vi "niScope Mux Open.vi"(8 "error in":errorcluster, 11 "adc session in":T2={"niScope"={"channel cfg"=[], "sessions"=[], "multi cards"=FALSE, "channels"=0, "type"=enum."n/a", "memory [B/chn]"=0, "ext. clock [Hz]"=0.0, "samples count"=0, "use streaming"=FALSE, "proc setup"={"packet size [smpl]"=0, "current timeout [s]"=0.0, "blk2blk timeout [s]"=0.0, "event time"=timestamp(0 s since 1904-01-01), "temp sampl T [s]"=0.0, "data queue"=refnum, "stop notifier"=refnum, "proc ref"=refnum}, "sample width [B]"=0, "ranges [V]"=[], "trigger setup"={"coupling"=1, "level [V]"=0.0, "slope"=0, "mode"=enum."Immediate"}, "fs [Hz]"=0.0, "bitres [bit]"=0, "clock source"=enum."VAL_NO_SOURCE"}, "3458A"={"channels"=[], "sync unit"={"VISA"="", "type"=enum."Picotest U6200A"}, "awg unit"={"type"=enum."Agilent 331xxA to 332xxA", "VISA"="", "enable 10MHz ref"=FALSE}, "sync mode"=enum."MASTER-SLAVE, MASTER clocked by TIMER", "streaming mode"=FALSE, "idn mode"=enum."Auto", "sampling mode"=enum."DCV", "Ts [s]"=0.0, "sample memory [B]"=0, "proc setup"={"channel id"=0, "packet size [smpl]"=0, "current timeout [s]"=0.0, "blk2blk timeout [s]"=0.0, "event time"=timestamp(0 s since 1904-01-01), "stop notifier"=refnum, "data queues"=[], "proc refs"=[], "bus semaphore"=refnum}, "sample size [B]"=0, "sample count"=0, "aux data"={"channel id"=0, "valid?"=[], "gain [V]"=[], "timestamp [s]"=[], "Ts [s]"=0.0, "abs timestamp"=timestamp(0 s since 1904-01-01), "t [deg C]"=[], "multiplex timestamp [s]"=-1.0, "only multiplex?"=FALSE, "multiplex smpl offset"=0}, "ranges [V]"=[], "aperture [s]"=0.0, "LEVEL trigger"={"edge"=enum."POS", "level [V]"=0.0, "coupling"=enum."DC"}, "trigger mode"=enum."AUTO", "measure temp.?"=FALSE, "disp mesages"=[], "shared bus?"=FALSE, "disable display?"=FALSE, "aper mode"=enum."Manual", "aper rules"=[], "multiplex"={"cycles"=0, "delay [s]"=0.0, "enabled"=FALSE, "overhead [s]"=1.0, "tot smpls"=0}}, "dsdll"={"dsdll"={"dsdll path"=path "", "dsdll handle"=[], "output devices"=[], "capture devices"=[]}, "channels"=0, "device id"=0, "channel idns"=[], "proc setup"={"packet size [smpl]"=0, "current timeout [s]"=0.0, "blk2blk timeout [s]"=0.0, "event time"=timestamp(0 s since 1904-01-01), "data queue"=refnum, "stop notifier"=refnum, "proc ref"=refnum}, "samples count"=0, "fs [Hz]"=0.0}, "type"=enum."niScope", "channel idn str"=[], "aux instr idn str"=[], "modified?"=FALSE, "simadc"={"channels"=[], "range [V]"=0.0, "Ts step [s]"=0.0, "time [s]"=0.0, "fs [Hz]"=0.0, "count"=0, "smpl offset"=0, "set count"=0, "bit res"=0}, "force rst?"=FALSE, "exit mode"=enum."Immediate reset", "exit dly"=0.0, "exit tmr"=timestamp(0 s since 1904-01-01), "busy?"=FALSE, "accessed?"=FALSE, "multiplex"={"Type"=enum."Dummy", "gen com ssn"={"visa"="", "primary"=enum."None", "secondary"=enum."None", "channels"=[]}, "delay before [s]"=0.0, "delay post [s]"=0.0, "sequence"=[], "enabled"=FALSE, "ref timestamp [s]"=0.0, "idn string"="", "dev niScope"="", "niScope idx"=0}} {"3458A"."channels"."Range [Vpk]" min=0.0; "niScope"."trigger setup"."level [V]" format="%.2f"; "niScope"."trigger setup"."coupling" items=["AC"=0, "DC"=1, "HF Reject"=3, "LF Reject"=4, "AC Plus HF Reject"=1001]; "niScope"."channel cfg"."Range [Vpk]" min=0.0; "niScope"."channel cfg"."Channel" min=0}) -> (0 "error out":errorcluster, 2 "idn string":string, 3 "adc session out":T2={"niScope"={"channel cfg"=[], "sessions"=[], "multi cards"=FALSE, "channels"=0, "type"=enum."n/a", "memory [B/chn]"=0, "ext. clock [Hz]"=0.0, "samples count"=0, "use streaming"=FALSE, "proc setup"={"packet size [smpl]"=0, "current timeout [s]"=0.0, "blk2blk timeout [s]"=0.0, "event time"=timestamp(0 s since 1904-01-01), "temp sampl T [s]"=0.0, "data queue"=refnum, "stop notifier"=refnum, "proc ref"=refnum}, "sample width [B]"=0, "ranges [V]"=[], "trigger setup"={"coupling"=1, "level [V]"=0.0, "slope"=0, "mode"=enum."Immediate"}, "fs [Hz]"=0.0, "bitres [bit]"=0, "clock source"=enum."VAL_NO_SOURCE"}, "3458A"={"channels"=[], "sync unit"={"VISA"="", "type"=enum."Picotest U6200A"}, "awg unit"={"type"=enum."Agilent 331xxA to 332xxA", "VISA"="", "enable 10MHz ref"=FALSE}, "sync mode"=enum."MASTER-SLAVE, MASTER clocked by TIMER", "streaming mode"=FALSE, "idn mode"=enum."Auto", "sampling mode"=enum."DCV", "Ts [s]"=0.0, "sample memory [B]"=0, "proc setup"={"channel id"=0, "packet size [smpl]"=0, "current timeout [s]"=0.0, "blk2blk timeout [s]"=0.0, "event time"=timestamp(0 s since 1904-01-01), "stop notifier"=refnum, "data queues"=[], "proc refs"=[], "bus semaphore"=refnum}, "sample size [B]"=0, "sample count"=0, "aux data"={"channel id"=0, "valid?"=[], "gain [V]"=[], "timestamp [s]"=[], "Ts [s]"=0.0, "abs timestamp"=timestamp(0 s since 1904-01-01), "t [deg C]"=[], "multiplex timestamp [s]"=-1.0, "only multiplex?"=FALSE, "multiplex smpl offset"=0}, "ranges [V]"=[], "aperture [s]"=0.0, "LEVEL trigger"={"edge"=enum."POS", "level [V]"=0.0, "coupling"=enum."DC"}, "trigger mode"=enum."AUTO", "measure temp.?"=FALSE, "disp mesages"=[], "shared bus?"=FALSE, "disable display?"=FALSE, "aper mode"=enum."Manual", "aper rules"=[], "multiplex"={"cycles"=0, "delay [s]"=0.0, "enabled"=FALSE, "overhead [s]"=1.0, "tot smpls"=0}}, "dsdll"={"dsdll"={"dsdll path"=path "", "dsdll handle"=[], "output devices"=[], "capture devices"=[]}, "channels"=0, "device id"=0, "channel idns"=[], "proc setup"={"packet size [smpl]"=0, "current timeout [s]"=0.0, "blk2blk timeout [s]"=0.0, "event time"=timestamp(0 s since 1904-01-01), "data queue"=refnum, "stop notifier"=refnum, "proc ref"=refnum}, "samples count"=0, "fs [Hz]"=0.0}, "type"=enum."niScope", "channel idn str"=[], "aux instr idn str"=[], "modified?"=FALSE, "simadc"={"channels"=[], "range [V]"=0.0, "Ts step [s]"=0.0, "time [s]"=0.0, "fs [Hz]"=0.0, "count"=0, "smpl offset"=0, "set count"=0, "bit res"=0}, "force rst?"=FALSE, "exit mode"=enum."Immediate reset", "exit dly"=0.0, "exit tmr"=timestamp(0 s since 1904-01-01), "busy?"=FALSE, "accessed?"=FALSE, "multiplex"={"Type"=enum."Dummy", "gen com ssn"={"visa"="", "primary"=enum."None", "secondary"=enum."None", "channels"=[]}, "delay before [s]"=0.0, "delay post [s]"=0.0, "sequence"=[], "enabled"=FALSE, "ref timestamp [s]"=0.0, "idn string"="", "dev niScope"="", "niScope idx"=0}} {"3458A"."channels"."Range [Vpk]" min=0.0; "niScope"."trigger setup"."level [V]" format="%.2f"; "niScope"."trigger setup"."coupling" items=["AC"=0, "DC"=1, "HF Reject"=3, "LF Reject"=4, "AC Plus HF Reject"=1001]; "niScope"."channel cfg"."Range [Vpk]" min=0.0; "niScope"."channel cfg"."Channel" min=0})   [LabVIEW 2013]
doc: "This VI tries to open virtual digitizer channel for multiplexer control. It shares device session with digitizer, so correct use is:\n1) initialize digitizer\n2) call this VI\n3) do stuff\n4) close multiplexer\n3) close digitizer"
uses:
  adc/ADC Session.ctl
  niScope/niScope Session.ctl
  niScope/niScope Virtual Channel Config.ctl
  niScope/niScope Virtual Channel Mode.ctl
  niScope/niScope Virtual Channel Input Z.ctl
  niScope/niScope Virtual Channel Coupling.ctl
  niScope/niScope Type.ctl
  niScope/niScope Digitizing Process Options.ctl
  niScope/niScope Data Packet.ctl
  niScope/niScope Trigger Setup.ctl
  <instrlib>/niScope/Controls/niScope trigger coupling.ctl
  <instrlib>/niScope/Controls/niScope trigger slope.ctl
  niScope/niScope Reference Clock.ctl
  DMM/3458A Digitizer Session.ctl
  DMM/3458A Virtual Channel Config.ctl
  Counter/Counter Session.ctl
  Counter/Counter Type.ctl
  AWG/AWG Session.ctl
  AWG/AWG Type.ctl
  DMM/3458A Sync Mode.ctl
  DMM/3458A Idn Mode.ctl
  DMM/3458A Digitizing Low Levels/Configure/Sampling Mode.ctl
  DMM/3458A Digitizing Process Options.ctl
  DMM/3458A Data Packet.ctl
  DMM/3458A Aux Record Data.ctl
  DMM/3458A Digitizing Low Levels/Configure/Level Setup.ctl
  DMM/3458A Digitizing Low Levels/Configure/First Sample Trigger.ctl
  DMM/3458A Aperture Selection Mode.ctl
  DMM/3458A Multiplexing Config.ctl
  dsdll/DSDLL Session.ctl
  dsdll/dsdll.lvlibp/dsdll_instance.ctl
  dsdll/dsdll.lvlibp/dsdll_device_record.ctl
  dsdll/DSDLL Process Config.ctl
  dsdll/DSDLL Data Packet.ctl
  adc/ADC Type.ctl
  simulated_adc/SimAdc Config.ctl
  simulated_adc/SimAdc Channel Cfg.ctl
  adc/ADC On Close Action.ctl
  adc/Multiplexer/MPX Session.ctl
  adc/Multiplexer/MPX Type.ctl
  Generic COM/GCOMM Session.ctl
  Generic COM/GCOMM Signal.ctl
  Generic COM/GCOMM Virtual Channel.ctl
  Generic COM/GCOMM Logic State.ctl
  <vilib>/Utility/error.llb/Error Cluster From Error Code.vi
  <vilib>/ErrorRing/Error Ring.xnode
  niScope/niScope Virtual Digitizer.lvlib
  DMM/3458A Virtual Digitizer.lvlib
  Counter/Counter.lvlib
  AWG/AWG.lvlib
  DMM/3458A Digitizing Low Levels/3458A Digitizing Low Levels.lvlib
  dsdll/dsdll.lvlibp
  dsdll/DSDLL Virtual Digitizer.lvlib
panel:
  in  "type":T1
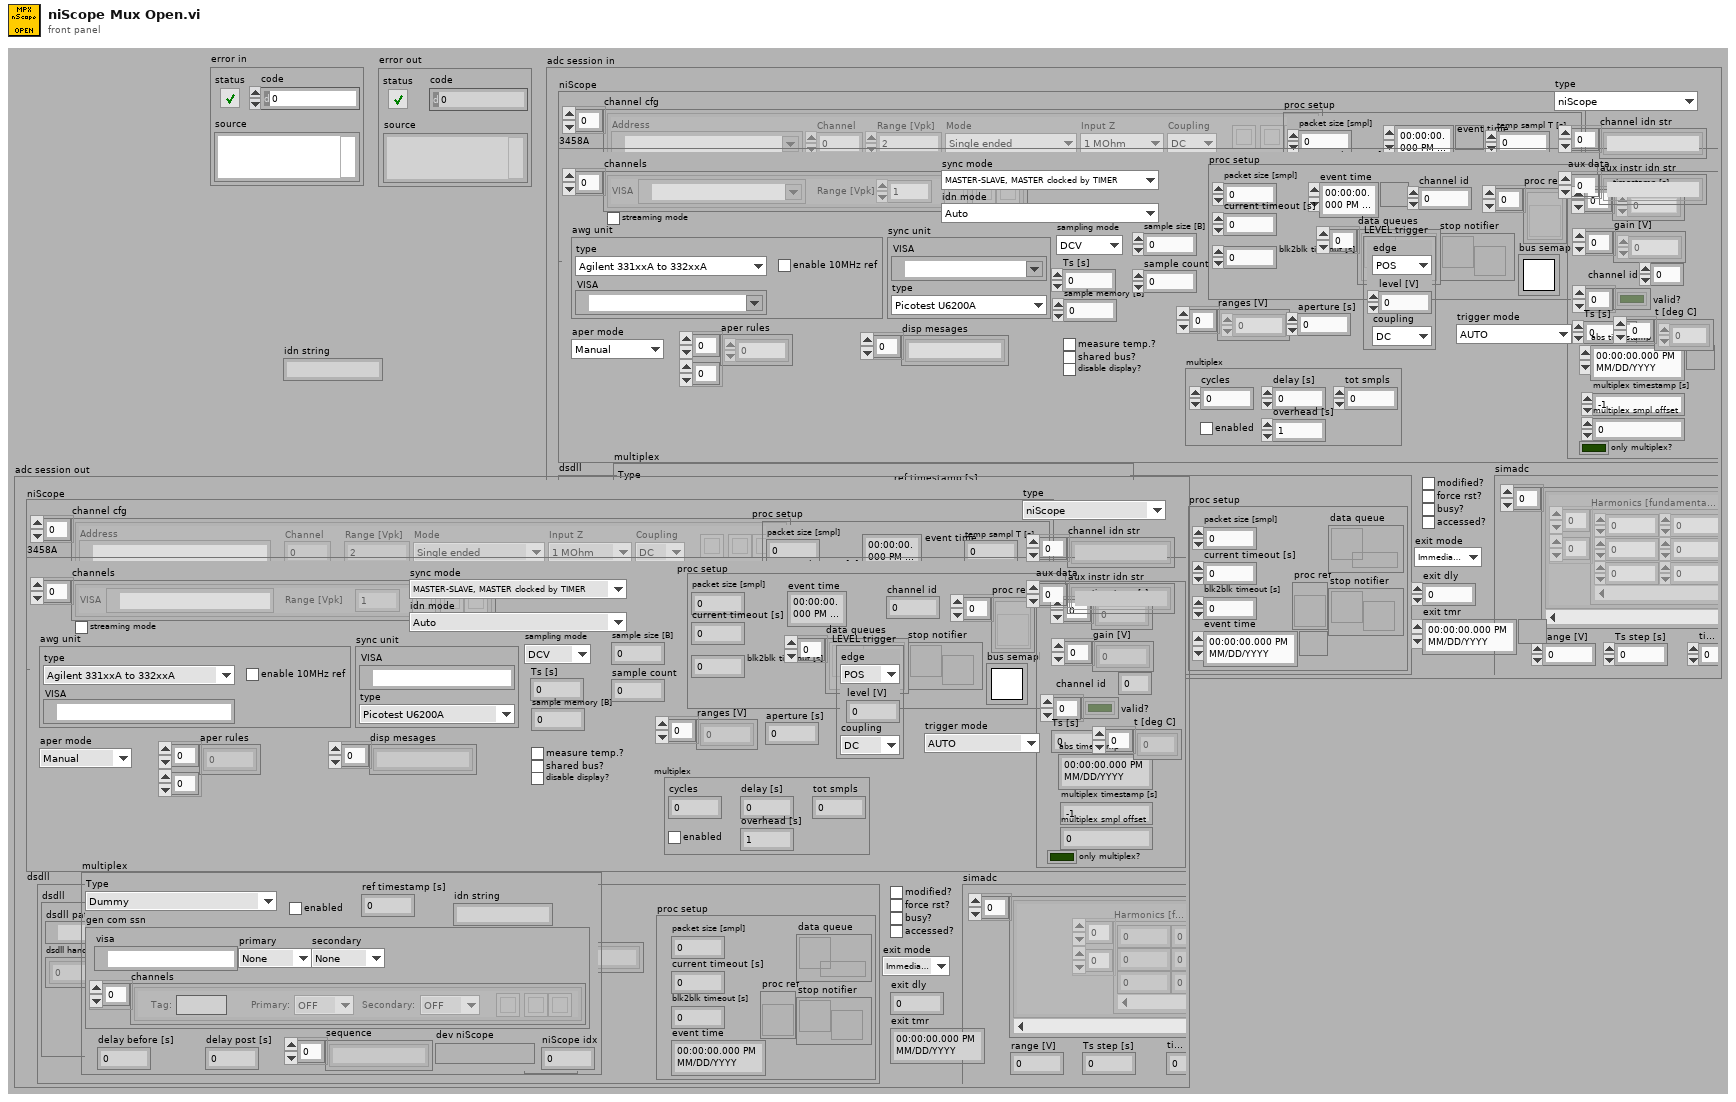
[diagram p1: front panel]
types:
  T1 = typedef "ADC Type.ctl" = enum16{"niScope", "3458A", "DirectSound DLL", "dummy"}
  T2 = typedef "ADC Session.ctl" = cluster{"niScope":T3, "3458A":T14, "dsdll":T30, "type":T1, "channel idn str":string[], "aux instr idn str":string[], "modified?":bool, "simadc":T34, "force rst?":bool, "exit mode":T36, "exit dly":dbl, "exit tmr":timestamp, "busy?":bool, "accessed?":bool, "multiplex":T37}
  T3 = typedef "niScope Virtual Digitizer.lvlib/niScope Session.ctl" = cluster{"channel cfg":T4[], "sessions":refnum<k20>[], "multi cards":bool, "channels":i32, "type":T8, "memory [B/chn]":i32, "ext. clock [Hz]":dbl, "samples count":i64, "use streaming":bool, "proc setup":T9, "sample width [B]":i32, "ranges [V]":dbl[], "trigger setup":T10, "fs [Hz]":dbl, "bitres [bit]":i32, "clock source":T13}
  T4 = typedef "niScope Virtual Digitizer.lvlib/niScope Virtual Channel Config.ctl" = cluster{"Address":refnum<k15>, "Channel":i32, "Mode":T5, "Input Z":T6, "Coupling":T7, "Range [Vpk]":dbl, "btn clr":bool, "btn up":bool, "btn down":bool}
  T5 = typedef "niScope Virtual Digitizer.lvlib/niScope Virtual Channel Mode.ctl" = enum16{"Single ended", "Unbal. differential", "Differential"}
  T6 = typedef "niScope Virtual Digitizer.lvlib/niScope Virtual Channel Input Z.ctl" = enum16{"1 MOhm", "50 Ohm"}
  T7 = typedef "niScope Virtual Digitizer.lvlib/niScope Virtual Channel Coupling.ctl" = enum16{"AC", "DC", "GND"}
  T8 = typedef "niScope Virtual Digitizer.lvlib/niScope Type.ctl" = enum16{"n/a", "5922"}
  T9 = typedef "niScope Virtual Digitizer.lvlib/niScope Digitizing Process Options.ctl" = cluster{"packet size [smpl]":i64, "current timeout [s]":dbl, "blk2blk timeout [s]":dbl, "event time":timestamp, "temp sampl T [s]":dbl, "data queue":refnum<queue>, "stop notifier":refnum<notifier>, "proc ref":refnum<vi>}
  T10 = typedef "niScope Virtual Digitizer.lvlib/niScope Trigger Setup.ctl" = cluster{"coupling":T11, "level [V]":dbl, "slope":T12, "mode":enum16{"Immediate", "External", "Level"}}
  T11 = typedef "niScope trigger coupling.ctl" = u16
  T12 = typedef "niScope trigger slope.ctl" = i32
  T13 = typedef "niScope Virtual Digitizer.lvlib/niScope Reference Clock.ctl" = enum16{"VAL_NO_SOURCE", "VAL_CLK_IN", "VAL_PXI_CLOCK", "VAL_EXTERNAL"}
  T14 = typedef "3458A Virtual Digitizer.lvlib/3458A Digitizer Session.ctl" = cluster{"channels":T15[], "sync unit":T16, "awg unit":T18, "sync mode":T20, "streaming mode":bool, "idn mode":T21, "sampling mode":T22, "Ts [s]":dbl, "sample memory [B]":i32, "proc setup":T23, "sample size [B]":i32, "sample count":i32, "aux data":T25, "ranges [V]":dbl[], "aperture [s]":dbl, "LEVEL trigger":T26, "trigger mode":T27, "measure temp.?":bool, "disp mesages":string[], "shared bus?":bool, "disable display?":bool, "aper mode":T28, "aper rules":dbl[][], "multiplex":T29}
  T15 = typedef "3458A Virtual Digitizer.lvlib/3458A Virtual Channel Config.ctl" = cluster{"VISA":refnum<visa-resource-name>, "Range [Vpk]":dbl, "btn clr":bool, "btn up":bool, "btn down":bool}
  T16 = typedef "Counter.lvlib/Counter Session.ctl" = cluster{"VISA":refnum<visa-resource-name>, "type":T17}
  T17 = typedef "Counter.lvlib/Counter Type.ctl" = enum16{"Picotest U6200A", "dummy"}
  T18 = typedef "AWG.lvlib/AWG Session.ctl" = cluster{"type":T19, "VISA":refnum<visa-resource-name>, "enable 10MHz ref":bool}
  T19 = typedef "AWG.lvlib/AWG Type.ctl" = enum16{"Agilent 331xxA to 332xxA", "Agilent 335xxA to 336xxA", "Tektronix AFG3101C", "dummy"}
  T20 = typedef "3458A Virtual Digitizer.lvlib/3458A Sync Mode.ctl" = enum16{"MASTER-SLAVE, MASTER clocked by TIMER", "MASTER-SLAVE, MASTER clocked by AWG", "ALL clocked by AWG", "MASTER-SLAVE, ALL clocked by TIMER", "ALL clocked by AWG with DFLL"}
  T21 = typedef "3458A Virtual Digitizer.lvlib/3458A Idn Mode.ctl" = enum16{"Auto", "Sequential (chn A, chn B, ...)", "From calibration string"}
  T22 = typedef "3458A Virtual Digitizer.lvlib/3458A Digitizing Low Levels.lvlib/Sampling Mode.ctl" = enum16{"DCV", "DSDC", "DSAC"}
  T23 = typedef "3458A Virtual Digitizer.lvlib/3458A Digitizing Process Options.ctl" = cluster{"channel id":i32, "packet size [smpl]":i32, "current timeout [s]":dbl, "blk2blk timeout [s]":dbl, "event time":timestamp, "stop notifier":refnum<notifier>, "data queues":refnum<queue>[], "proc refs":refnum<vi>[], "bus semaphore":T24}
  T24 = typedef "Semaphore RefNum" = refnum<k1>
  T25 = typedef "3458A Virtual Digitizer.lvlib/3458A Aux Record Data.ctl" = cluster{"channel id":i32, "valid?":bool[], "gain [V]":dbl[], "timestamp [s]":dbl[], "Ts [s]":dbl, "abs timestamp":timestamp, "t [deg C]":dbl[], "multiplex timestamp [s]":dbl, "only multiplex?":bool, "multiplex smpl offset":i64}
  T26 = typedef "3458A Virtual Digitizer.lvlib/3458A Digitizing Low Levels.lvlib/Level Setup.ctl" = cluster{"edge":enum16{"POS", "NEG"}, "level [V]":dbl, "coupling":enum16{"DC", "AC"}}
  T27 = typedef "3458A Virtual Digitizer.lvlib/3458A Digitizing Low Levels.lvlib/First Sample Trigger.ctl" = enum16{"AUTO", "EXT", "SYN", "SGL", "HOLD", "LEVEL"}
  T28 = typedef "3458A Virtual Digitizer.lvlib/3458A Aperture Selection Mode.ctl" = enum16{"Manual", "Maximum", "Table"}
  T29 = typedef "3458A Multiplexing Config.ctl" = cluster{"cycles":i32, "delay [s]":dbl, "enabled":bool, "overhead [s]":dbl, "tot smpls":i64}
  T30 = typedef "DSDLL Virtual Digitizer.lvlib/DSDLL Session.ctl" = cluster{"dsdll":T31, "channels":i32, "device id":i32, "channel idns":string[], "proc setup":T33, "samples count":i32, "fs [Hz]":dbl}
  T31 = typedef "dsdll.lvlibp/dsdll_instance.ctl" = cluster{"dsdll path":path, "dsdll handle":u8[], "output devices":T32[], "capture devices":T32[]}
  T32 = typedef "dsdll.lvlibp/dsdll_device_record.ctl" = cluster{"guid":u8[], "name":string}
  T33 = typedef "DSDLL Virtual Digitizer.lvlib/DSDLL Process Config.ctl" = cluster{"packet size [smpl]":i32, "current timeout [s]":dbl, "blk2blk timeout [s]":dbl, "event time":timestamp, "data queue":refnum<queue>, "stop notifier":refnum<notifier>, "proc ref":refnum<vi>}
  T34 = typedef "SimAdc Config.ctl" = cluster{"channels":T35[], "range [V]":dbl, "Ts step [s]":dbl, "time [s]":dbl, "fs [Hz]":dbl, "count":i64, "smpl offset":i64, "set count":i64, "bit res":i32}
  T35 = typedef "SimAdc Channel Cfg.ctl" = cluster{"harmonics":dbl[][], "btn clear":bool, "noise":dbl, "fundamental [Hz]":dbl}
  T36 = typedef "ADC On Close Action.ctl" = enum16{"Immediate reset", "Delayed reset"}
  T37 = typedef "MPX Session.ctl" = cluster{"Type":T38, "gen com ssn":T39, "delay before [s]":dbl, "delay post [s]":dbl, "sequence":string[], "enabled":bool, "ref timestamp [s]":dbl, "idn string":string, "dev niScope":refnum<k15>, "niScope idx":i32}
  T38 = typedef "MPX Type.ctl" = enum16{"Dummy", "Generic - COM port", "Generic - niScope PFI"}
  T39 = typedef "GCOMM Session.ctl" = cluster{"visa":refnum<visa-resource-name>, "primary":T40, "secondary":T40, "channels":T41[]}
  T40 = typedef "GCOMM Signal.ctl" = enum16{"None", "DTR", "RTS"}
  T41 = typedef "GCOMM Virtual Channel.ctl" = cluster{"Primary:":T42, "Secondary:":T42, "btn clr":bool, "btn up":bool, "btn down":bool, "Tag:":string}
  T42 = typedef "GCOMM Logic State.ctl" = enum16{"OFF", "ON"}
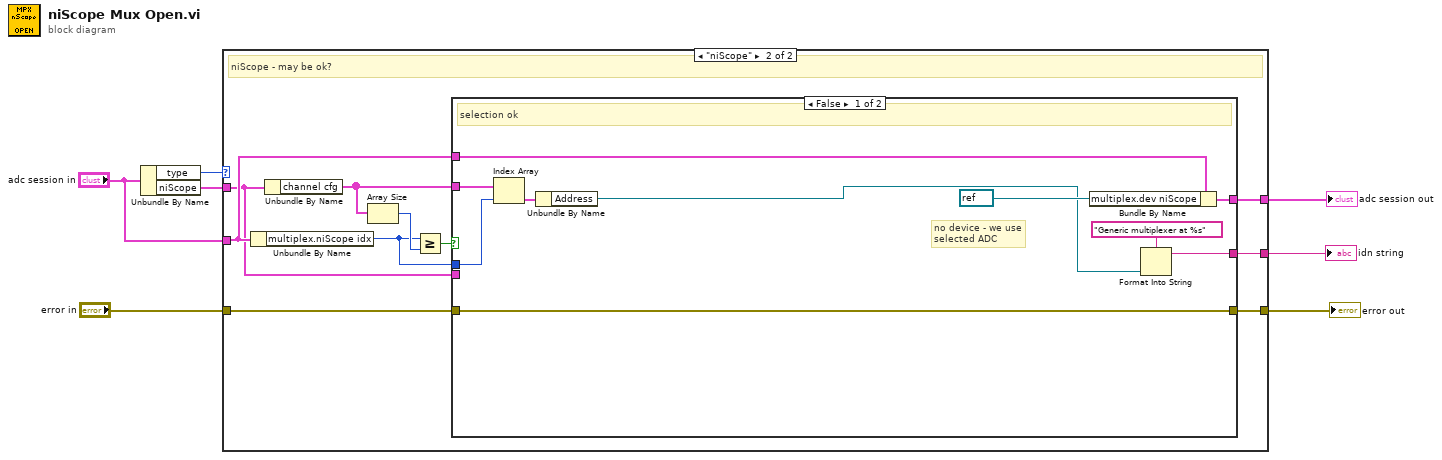
[diagram p0: block diagram]
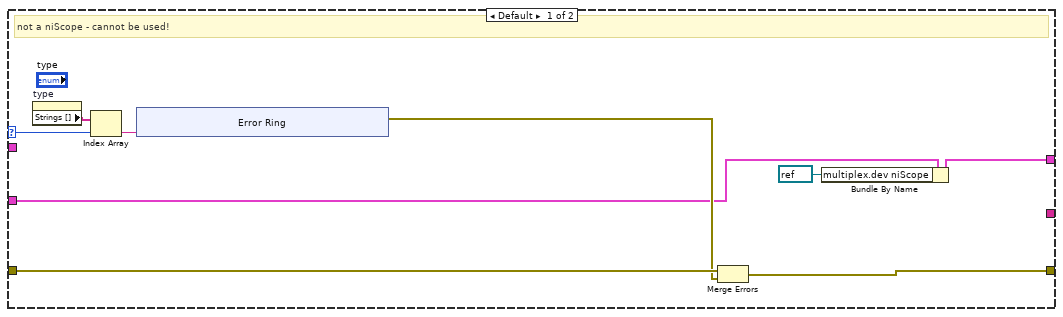
[diagram p2: hidden frame]
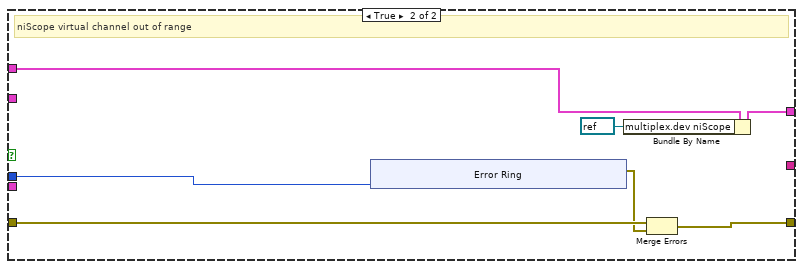
[diagram p3: hidden frame]
diagram:
  n1 = Unbundle By Name("adc session in") -> ("type"=w7:T1, "niScope"=w4:T3)
  n2 = case shown="\"niScope\"" w7 {
    selector: w7 -> [w15 _]
    tunnel: "error in" -> [w13 w30]
    tunnel: [w11 w29] -> w5
    tunnel: w4 -> [_ w24]
    tunnel: "adc session in" -> [w10 w27]
    tunnel: [_ w26] -> w2
    tunnel: [w9 w25] -> w1
    frame Default {
      # "not a niScope - cannot be used!"
      n3 = property on="type" class="Enum (strict)"() -> ("Strings []"=w16:string[])  [unwired: 2 in, 2 out]
      n4 = Index Array(array=w16, index=w15) -> (element=w14:string)
      n5 = xnode "Error Ring"("parameter 0"=w14) -> ("error out"=w12:errorcluster)
      n6 = Merge Errors(w13, w12) -> (w11:errorcluster)
      n7 = Bundle By Name(cluster=w10, "multiplex.dev niScope"=refnum<k15> refnum) -> (w9:T2)
    }
    frame "niScope" {
      # "niScope - may be ok?"
      n8 = Unbundle By Name(w27) -> ("multiplex.niScope idx"=w31:i32)
      n9 = Unbundle By Name(w24) -> ("channel cfg"=w28:T4[])
      n10 = Array Size(array=w28) -> (size(s)=w33:i32)
      n11 = Greater Or Equal?(x=w31, y=w33) -> (x >= y?=w32:bool)
      n12 = case shown="False" w32 {
        tunnel: w31 -> [w42 w50]
        tunnel: w30 -> [w34 w49]
        tunnel: [w34 w47] -> w29
        tunnel: w28 -> [w43 _]
        tunnel: w27 -> [w40 w46]
        tunnel: [w38 _] -> w26
        tunnel: [w37 w45] -> w25
        tunnel: w24 -> [_ _]
        frame False {
          # "no device - we use\nselected ADC"
          # "selection ok"
          n13 = Index Array(array=w43, index=w42) -> (element=w41:T4)
          n14 = Unbundle By Name(w41) -> ("Address"=w35:refnum<k15>)
          n15 = Bundle By Name(cluster=w40, "multiplex.dev niScope"=refnum<k15> refnum ("reference out")) -> (w37:T2)
          n16 = Format Into String(format string="Generic multiplexer at %s", w35) -> (resulting string=w38:string)  [unwired: 2 in, 1 out]
        }
        frame True {
          # "niScope virtual channel out of range"
          n17 = xnode "Error Ring"("parameter 0"=w50) -> ("error out"=w48:errorcluster)
          n18 = Bundle By Name(cluster=w46, "multiplex.dev niScope"=refnum<k15> refnum) -> (w45:T2)
          n19 = Merge Errors(w49, w48) -> (w47:errorcluster)
        }
      }
    }
  }
  "error out" <- w5
  "adc session out" <- w1
  "idn string" <- w2
